vi "Get_Speed.vi"(8 "error in (no error)":errorcluster, 11 "Lifter_motor in":refnum<class "Lifter_motor.lvclass">) -> (0 "error out":errorcluster, 1 "Motor Speed (rev/s)":dbl, 2 "Target Velocity (mm/s)":dbl, 3 "Lifter_motor out":refnum<class "Lifter_motor.lvclass">)   [LabVIEW 2019, in "Lifter_motor.lvclass"]
uses:
  Lifter_motor.lvclass
  Lifter_motor.lvclass/Lifter_motor.ctl
  TCP Class/LifterTCP.lvclass
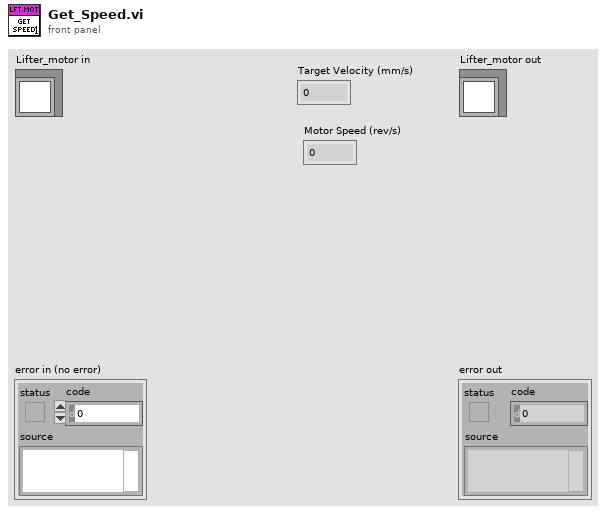
[diagram p1: front panel]
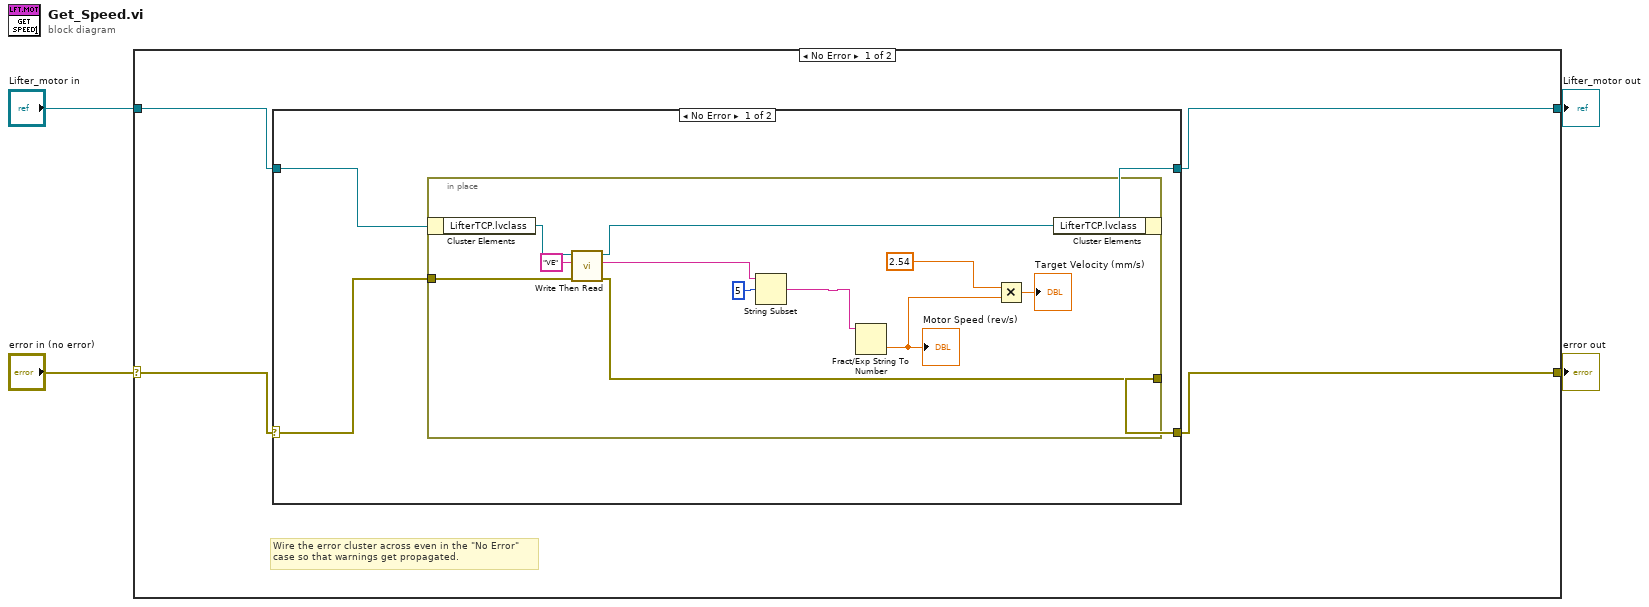
[diagram p0: block diagram]
diagram:
  n1 = case shown="No Error" "error in (no error)" {
    selector: "error in (no error)" -> [w7 w27]
    tunnel: [w6 w27] -> w3
    tunnel: [w5 w26] -> w1
    tunnel: "Lifter_motor in" -> [w8 w26]
    frame No Error {
      # "Wire the error cluster across even in the \"No Error\"\ncase so that warnings get propagated."
      n2 = case shown="No Error" w7 {
        selector: w7 -> [w10 w25]
        tunnel: [w9 w25] -> w6
        tunnel: [w11 w24] -> w5
        tunnel: w8 -> [w12 w24]
        frame No Error {
          n3 = in-place {
            in-place-border: w10 -> [w22]
            in-place-border: [w18] -> w9
            n4 = in-place-cluster #1(w12) -> ("LifterTCP.lvclass"=w23:refnum<class "LifterTCP.lvclass">)
            n5 = call "Write Then Read.vi"("error in (no error)"=w22, "Parameter 1"="VE", "LifterTCP in"=w23) -> ("error out"=w18:errorcluster, "Read Data"=w20:string, "LifterTCP out"=w19:refnum<class "LifterTCP.lvclass">)  [unwired: 6 in]
            n6 = String Subset(string=w20, offset (0)=5) -> (substring=w14:string)  [unwired: 1 in]
            n7 = Fract/Exp String To Number(string=w14) -> (number=w13:dbl)  [unwired: 3 in, 1 out]
            "Motor Speed (rev/s)" <- w13
            n8 = Multiply(x=2.54, y=w13) -> (x*y=→"Target Velocity (mm/s)":dbl)
            n9 = in-place-cluster #1("LifterTCP.lvclass"=w19) -> (w11:refnum<class "Lifter_motor.lvclass">)
          }
        }
        frame Error {
        }
      }
    }
    frame Error {
    }
  }
  "error out" <- w3
  "Lifter_motor out" <- w1
